vi "Calculate Trend.vi"(9 "WaveformGraph in":refnum<vi>, 10 "Display State In in":T1 caption="State", 11 "Data In in":T3) -> (2 "Display State In out":T1 caption="State", 3 "Data In out":T3)   [LabVIEW 2015, in "XTrend.xctl"]
uses:
  XTrend.xctl
  XTrend_Data.ctl
  XTrend_State.ctl
  View Mode.ctl
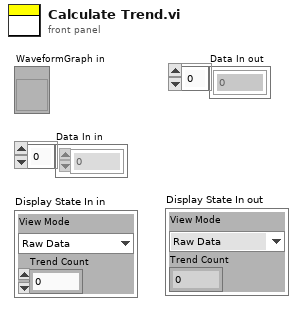
[diagram p1: front panel]
types:
  T1 = typedef "XTrend.xctl/XTrend_State.ctl" = cluster{"View Mode":T2, "Trend Count":dbl}
  T2 = typedef "View Mode.ctl" = enum16{"Raw Data", "Trend"}
  T3 = typedef "XTrend.xctl/XTrend_Data.ctl" = dbl[]
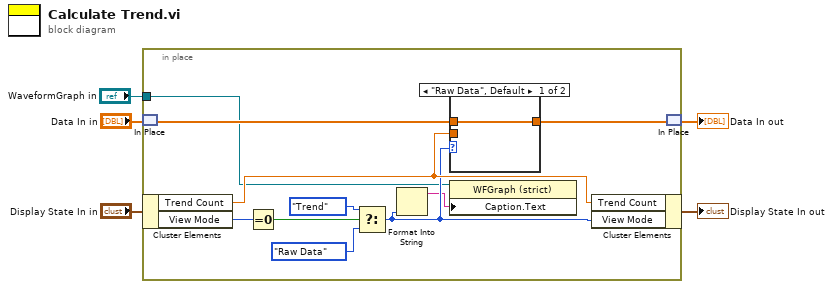
[diagram p0: block diagram]
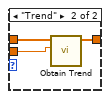
[diagram p2: hidden frame]
diagram:
  n1 = in-place {
    in-place-border: "WaveformGraph in" -> [w7]
    n2 = in-place-match #1("Data In in") -> (w15:T3)
    n3 = in-place-cluster #2("Display State In in") -> ("Trend Count"=w13:dbl, "View Mode"=w12:T2)
    n4 = Equal To 0?(x=w12) -> (x = 0?=w11:bool)
    n5 = Select(t=View_Mode."Trend" ("View Mode"), s=w11, f=View_Mode."Raw Data" ("View Mode")) -> (s? t:f=w8:T2)
    n6 = Format Into String(w8) -> (resulting string=w6:string)  [unwired: 3 in, 1 out]
    n7 = case shown="\"Raw Data\", Default" w8 {
      tunnel: w15 -> [w16 w19]
      tunnel: [w16 w18] -> w14
      tunnel: w13 -> [_ w17]
      frame "Raw Data", Default {
      }
      frame "Trend" {
        n8 = call "Obtain Trend.vi"("Trend Count"=w17, "Data In"=w19) -> ("Array"=w18:dbl[])  [unwired: 9 in]
      }
    }
    n9 = property class="WFGraph (strict)"(reference=w7, "Caption.Text"=w6) -> ()  [unwired: 1 in, 2 out]
    n10 = in-place-cluster #2("Trend Count"=w13, "View Mode"=w8) -> (→"Display State In out":T1)
    n11 = in-place-match #1(w14) -> (→"Data In out":T3)
  }
